vi "Read Max V.vi"(8 "error in (no error)":errorcluster, 11 "Acopian in":refnum<class "Acopian.lvclass">) -> (0 "error out":errorcluster, 2 "Max V":dbl, 3 "Acopian out":refnum<class "Acopian.lvclass">)   [LabVIEW 2019, in "Acopian.lvlib" / "Acopian.lvclass"]
uses:
  Library/Acopian.lvclass
  Library/Acopian.lvclass/Acopian.ctl
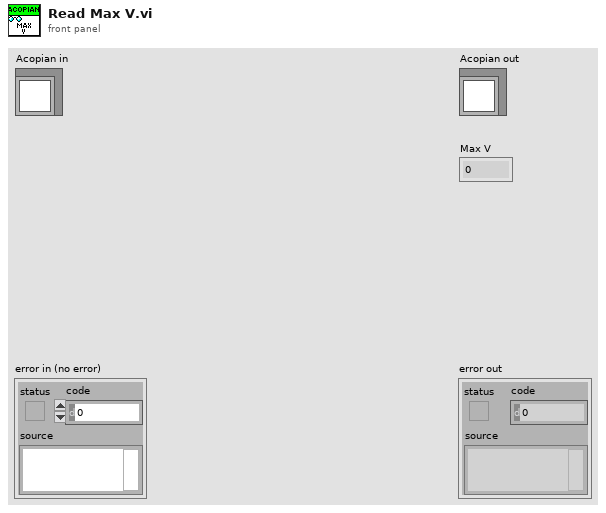
[diagram p1: front panel]
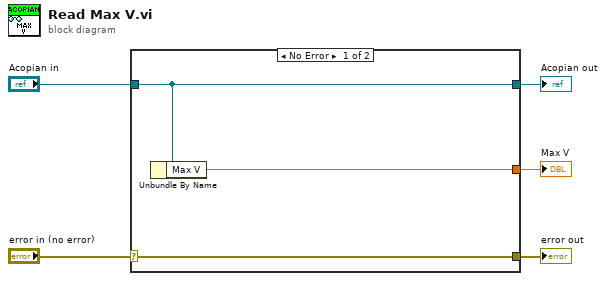
[diagram p0: block diagram]
diagram:
  n1 = case shown="No Error" "error in (no error)" {
    selector: "error in (no error)" -> [w8 w9]
    tunnel: [w8 w9] -> w4
    tunnel: [w7 w10] -> w2
    tunnel: "Acopian in" -> [w7 w10]
    tunnel: [w6 _] -> w1
    frame No Error {
      n2 = Unbundle By Name(w7) -> ("Max V"=w6:dbl)
    }
    frame Error {
    }
  }
  "error out" <- w4
  "Acopian out" <- w2
  "Max V" <- w1
